vi "Get Joystick Axis Target.vi"(8 "error in (no error)":errorcluster, 9 "Joystick Device Number":string, 10 "Joystick Axis Number (1)":i32=1, 11 "VISA resource name":refnum<visa-resource-name>) -> (0 "error out":errorcluster, 1 "Target Axis Number":i32, 2 "Target Device Number":i32, 3 "VISA resource name out":refnum<visa-resource-name>, 4 "Target Axis Type":u16(ring)=1 items=["axis", "lockstep group", "virtual axis"])   [LabVIEW 2015, in "Zaber A Series.lvlib"]
doc: "Use this VI to determine what device and axis are targeted by a particular joystick axis. \n\nInput the device number of the joystick to query and the number of the axis to check - 1 is the X axis, 2 is Y and 3 is the rotation of the knob on the end of the joystick.\n\nThe output is the device number and axis number targeted by the specified joystick axis, and what type of axis the joystick thinks it is (normal, lockstep group or virtual axis)."
uses:
  Zaber A Series.lvlib
  Private/All Commands.ctl
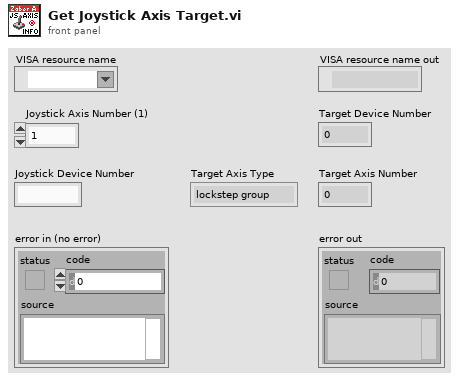
[diagram p1: front panel]
types:
  T1 = typedef "Zaber A Series.lvlib/All Commands.ctl" = string
  T2 = cluster{"Device":string, "Axis":string, "Reply Flag":string, "Status":string, "Warning Flags":string, "Data":string}
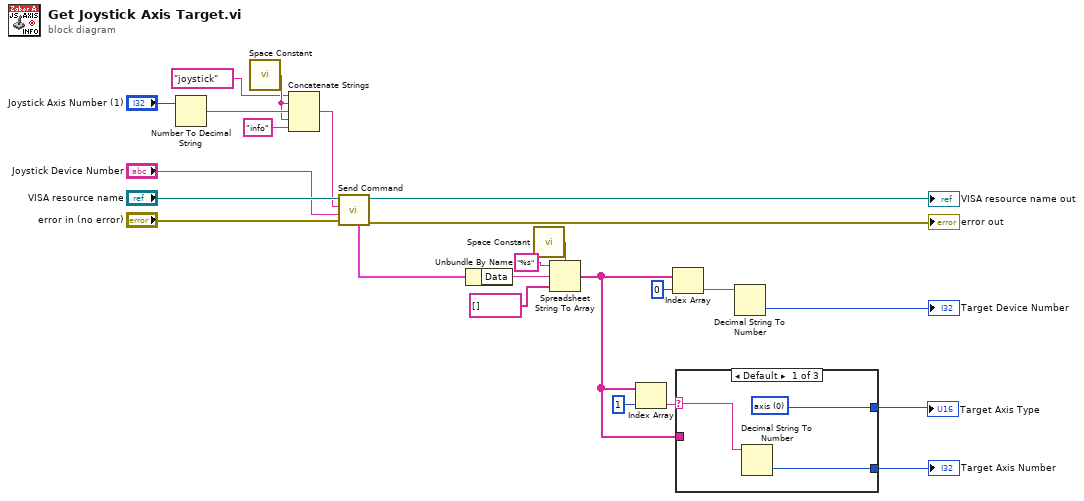
[diagram p0: block diagram]
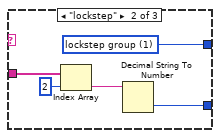
[diagram p2: hidden frame]
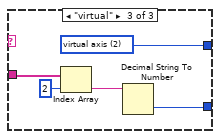
[diagram p3: hidden frame]
diagram:
  n1 = Number To Decimal String(number="Joystick Axis Number (1)") -> (decimal integer string=w21:string)  [unwired: 1 in]
  n2 = call <vilib>:"Space Constant.vi"() -> ("String"=w20:string)
  n3 = Concatenate Strings(T1 "joystick" ("Complete Command List"), w20, w21, w20, "info" ("string")) -> (w18:string)
  n4 = call "Send Command.vi"("error in (no error)"="error in (no error)", "Device and Axis"="Joystick Device Number", "Command"=w18, "VISA resource name"="VISA resource name") -> ("error out"=→"error out":errorcluster, "VISA resource name out"=→"VISA resource name out":refnum<visa-resource-name>, "First Response Bundle"=w1:T2)  [unwired: 2 in, 3 out]
  n5 = Unbundle By Name(w1) -> ("Data"=w16:string)
  n6 = call <vilib>:"Space Constant.vi"() -> ("String"=w14:string)
  n7 = Spreadsheet String To Array(delimiter (Tab)=w14, format string="%s", spreadsheet string=w16, array type (2D Dbl)=string[] []) -> (array=w6:string[])
  n8 = Index Array(array=w6, index=1) -> (element=w8:string)
  n9 = Index Array(array=w6, index=0) -> (element=w11:string)
  n10 = case shown="Default" w8 {
    selector: w8 -> [w27 _ _]
    tunnel: [w26 w29 w34] -> w7
    tunnel: w6 -> [_ w32 w35]
    tunnel: [w25 w28 w33] -> w2
    frame Default {
      w25 = u16 0 items=["axis", "lockstep group", "virtual axis"]
      n11 = Decimal String To Number(string=w27) -> (number=w26:i32)  [unwired: 2 in, 1 out]
    }
    frame "lockstep" {
      w28 = u16 1 items=["axis", "lockstep group", "virtual axis"]
      n12 = Index Array(array=w32, index=2) -> (element=w30:string)
      n13 = Decimal String To Number(string=w30) -> (number=w29:i32)  [unwired: 2 in, 1 out]
    }
    frame "virtual" {
      w33 = u16 2 items=["axis", "lockstep group", "virtual axis"]
      n14 = Index Array(array=w35, index=2) -> (element=w37:string)
      n15 = Decimal String To Number(string=w37) -> (number=w34:i32)  [unwired: 2 in, 1 out]
    }
  }
  "Target Axis Number" <- w7
  "Target Axis Type" <- w2
  n16 = Decimal String To Number(string=w11) -> (number=→"Target Device Number":i32)  [unwired: 2 in, 1 out]
